vi "Configure.vi"(8 "error in (no error)":errorcluster, 11 "QuickNote in":refnum<class "QuickNote.lvclass">) -> (0 "error out":errorcluster, 3 "QuickNote out":refnum<class "QuickNote.lvclass">)   [LabVIEW 2020, in "QuickNote.lvlib" / "QuickNote.lvclass"]
uses:
  QuickNote.lvclass
  DataProcessor/DataProcessor/DataProcessor.lvclass
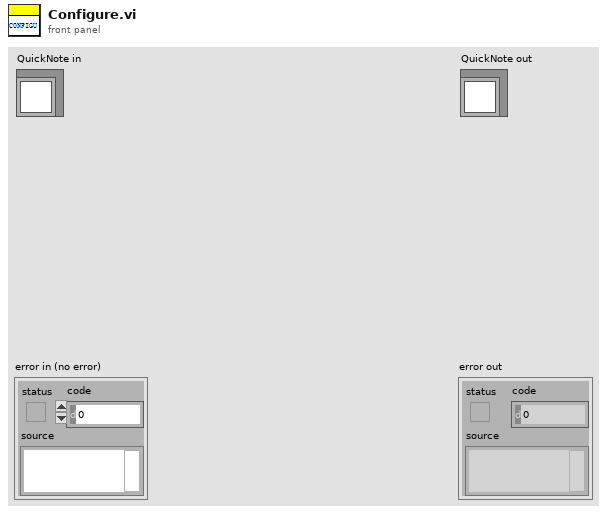
[diagram p1: front panel]
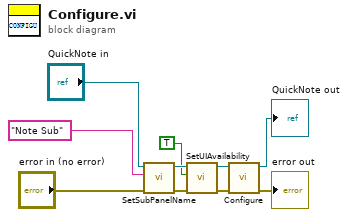
[diagram p0: block diagram]
diagram:
  n1 = call-dynamic "SetSubPanelName.vi"("error in (no error)"="error in (no error)", "Panel"="Note Sub", "DataProcessor in"="QuickNote in") -> ("error out"=w7:errorcluster, "DataProcessor out"=w3:refnum<class "QuickNote.lvclass">)  [unwired: 7 in]
  n2 = call-dynamic "SetUIAvailability.vi"("error in (no error)"=w7, "HasUI?"=TRUE ("Has UI?(T)"), "DataProcessor in"=w3) -> ("error out"=w4:errorcluster, "DataProcessor out"=w2:refnum<class "QuickNote.lvclass">)  [unwired: 7 in]
  n3 = call-parent "Configure.vi"("error in (no error)"=w4, "DataProcessor in"=w2) -> ("error out"=→"error out":errorcluster, "DataProcessor out"=→"QuickNote out":refnum<class "QuickNote.lvclass">)  [unwired: 8 in]
